vi "File handler.vi"(1 "Path in":path, 2 "Default file name":string, 3 "Read (F) or write (T)?":bool, 4 "Write new File?":bool, 6 "Extension":string="txt", 7 "With dialog?":bool) -> (14 "Path out":path, 15 "Cancelled?":bool, 16 "Data added?":bool)   [LabVIEW 2020]
doc: "This VI handles file name selections with or without a user interface. Files can be read or written. Path in is the path to the file to read or write. Extension is the file extension for the file to write (e.g. txt, jpg). If Read (F) or write (T) is TRUE, Extension must be given and entry must not have a dot. If With dialog? is TRUE, in every case a dialog box will pop up where the file to read or write can be selected. Default file name is used for naming suggestions if a dialog pops up. If Read (F) or write (T)? is TRUE and Write new file? is TRUE, a dialog box will pop up if the selected file name already exists. If Write new file? is FALSE and the selected file name already exists, a dialog box will pop up to ask if data should be added. Data added? indicates if data was added to an existing file. Cancelled? indicates if the user has cancelled the operation. Path out is NotAPath if operation was cancelled or not successful and contains the selected path for the file which was read or written if the operation was successful."
panel:
  # "This vi handles file name selections with or without a user interface.\nFor file writing, \"Extension\" must be given and entry must not have a dot.\nSee manual or VI description for more information."
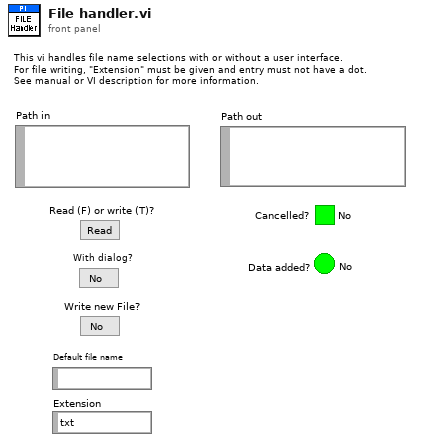
[diagram p1: front panel]
types:
  T1 = enum32{"existing file", "new file", "new or existing file", "existing dir", "new dir", "new or existing dir", "existing file (use LLBs)", "new file (use LLBs)", "new or existing file (use LLBs)", "new or existing file or directory (use LLBs)"}
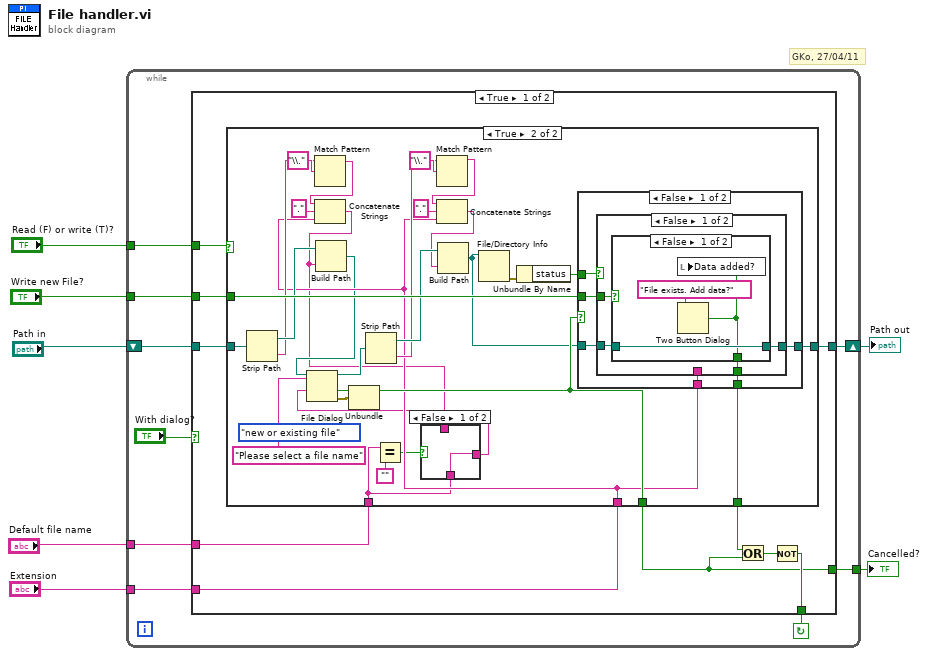
[diagram p0: block diagram]
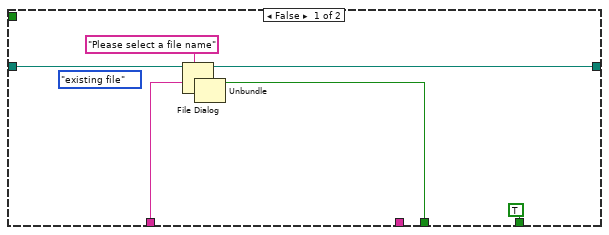
[diagram p2: hidden frame]
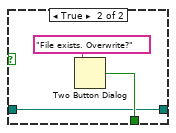
[diagram p4: hidden frame]
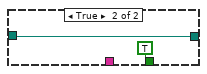
[diagram p5: hidden frame]
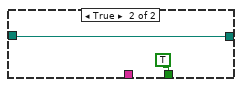
[diagram p6: hidden frame]
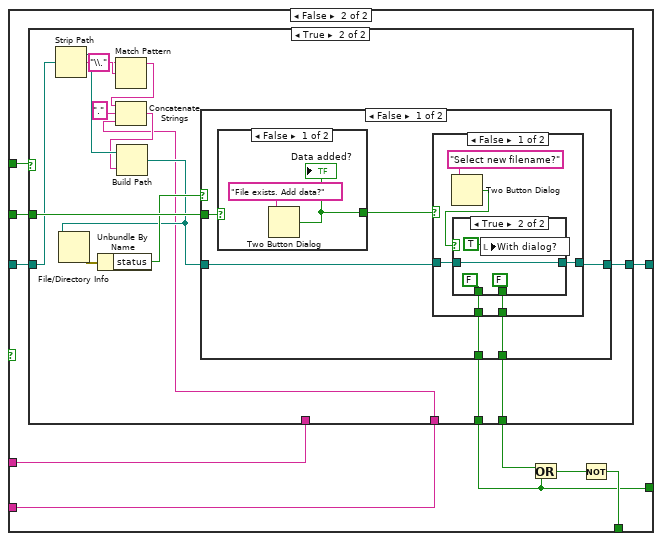
[diagram p7: hidden frame]
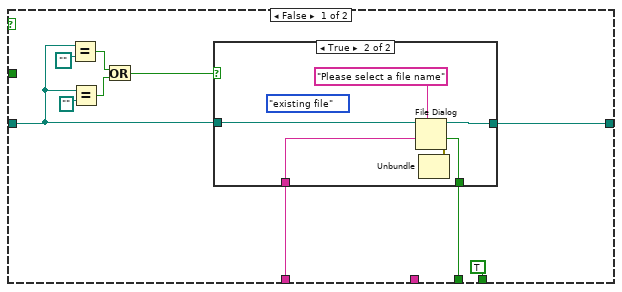
[diagram p8: hidden frame]
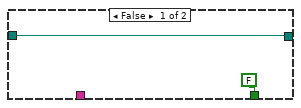
[diagram p9: hidden frame]
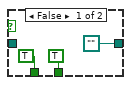
[diagram p10: hidden frame]
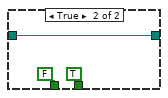
[diagram p11: hidden frame]
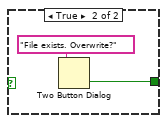
[diagram p12: hidden frame]
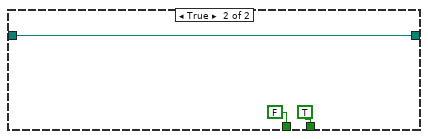
[diagram p13: hidden frame]
diagram:
  # "GKo, 27/04/11"
  n1 = while {
    tunnel: "Extension" -> [w9]
    shift-left: "Path in" -> [w10]
    shift-right: [w11] -> w3
    tunnel: "Default file name" -> [w12]
    tunnel: "Read (F) or write (T)?" -> [w14]
    tunnel: "Write new File?" -> [w15]
    tunnel: [w13] -> w6
    stop <- w16 continue-if-true
    n2 = case shown="True" "With dialog?" {
      tunnel: [w24 w92] -> w16
      tunnel: w15 -> [w23 w91]
      tunnel: w14 -> [w22 w90]
      tunnel: [w18 w86] -> w13
      tunnel: [w21 w89] -> w11
      tunnel: w10 -> [w19 w87]
      tunnel: w12 -> [w20 w88]
      tunnel: w9 -> [w17 w85]
      frame True {
        n3 = case shown="True" w22 {
          tunnel: [TRUE ("T button?") w62] -> w26
          tunnel: w23 -> [_ w61]
          tunnel: [w32 w58] -> w18
          tunnel: [w30 w60] -> w21
          tunnel: w20 -> [w29 w36]
          tunnel: w19 -> [w31 w52]
          tunnel: w17 -> [_ w44]
          frame False {
            (unwired) T1."existing file" ("select mode (2)")
            n4 = File Dialog(7:"Please select a file name" ("prompt"), 9:w29, 11:w31) -> (0:w27:errorcluster, 1:w32:bool, 3:w30:path)  [unwired: 1 in, 4 out]
            n5 = Unbundle(w27) -> ()  [unwired: 3 out]
          }
          frame True {
            (unwired) T1."new or existing file" ("select mode (2)")
            n6 = Strip Path(path=w52) -> (stripped path=w56:path, name=w55:string)
            n7 = Match Pattern(string=w55, regular expression="\\." ("search char (-)")) -> (before substring=w54:string)  [unwired: 4 out]
            n8 = Concatenate Strings(w54, "." ("Substring"), w44) -> (w37:string)
            n9 = Build Path(base path=w56, name or relative path=w37) -> (appended path=w43:path)
            n10 = Equal?(x=w36, y="") -> (x = y?=w38:bool)
            n11 = case shown="False" w38 {
              tunnel: [w63 w64] -> w35
              tunnel: w37 -> [_ w64]
              tunnel: w36 -> [w63 _]
              frame False {
              }
              frame True {
              }
            }
            n12 = File Dialog(7:"Please select a file name" ("prompt"), 9:w35, 11:w43) -> (0:w34:errorcluster, 1:w58:bool, 3:w47:path)  [unwired: 1 in, 4 out]
            n13 = Unbundle(w34) -> ()  [unwired: 3 out]
            n14 = Strip Path(path=w47) -> (stripped path=w50:path, name=w49:string)
            n15 = Match Pattern(string=w49, regular expression="\\." ("search char (-)")) -> (before substring=w46:string)  [unwired: 4 out]
            n16 = Concatenate Strings(w46, "." ("Substring"), w44) -> (w45:string)
            n17 = Build Path(base path=w50, name or relative path=w45) -> (appended path=w42:path)
            n18 = File/Directory Info(path=w42) -> (error out=w41:errorcluster)  [unwired: 1 in, 6 out]
            n19 = Unbundle By Name(w41) -> ("status"=w40:bool)
            n20 = case shown="False" w58 {
              tunnel: [w70 TRUE ("T button?")] -> w62
              tunnel: w61 -> [w69 _]
              tunnel: w40 -> [w68 _]
              tunnel: w42 -> [w67 w83]
              tunnel: [w66 w83] -> w60
              tunnel: w44 -> [w65 _]
              frame False {
                n21 = case shown="False" w68 {
                  tunnel: [w74 TRUE] -> w70
                  tunnel: w69 -> [w73 _]
                  tunnel: w67 -> [w71 w81]
                  tunnel: [w72 w81] -> w66
                  tunnel: w65 -> [_ _]
                  frame False {
                    n22 = case shown="False" w73 {
                      tunnel: [w75 w79] -> w74
                      tunnel: [w76 w78] -> w72
                      tunnel: w71 -> [w76 w78]
                      frame False {
                        n23 = Two Button Dialog(message="File exists. Add data?") -> (T button?=w75:bool)  [unwired: 2 out]
                        n24 = local write "Data added?"(w75) -> ()
                      }
                      frame True {
                        n25 = Two Button Dialog(message="File exists. Overwrite?") -> (T button?=w79:bool)  [unwired: 2 out]
                      }
                    }
                  }
                  frame True {
                  }
                }
              }
              frame True {
              }
            }
          }
        }
        n26 = Or(x=w26, y=w18) -> (x .or. y?=w25:bool)
        n27 = Not(x=w25) -> (.not. x?=w24:bool)
      }
      frame False {
        n28 = case shown="True" w90 {
          tunnel: [TRUE ("T button?") w127] -> w94
          tunnel: w91 -> [_ w126]
          tunnel: [w104 w115] -> w86
          tunnel: [w103 w125] -> w89
          tunnel: w88 -> [w102 _]
          tunnel: w87 -> [w98 w118]
          tunnel: w85 -> [_ w113]
          frame False {
            n29 = Equal?(x=w98, y=path "") -> (x = y?=w96:bool)
            n30 = Equal?(x=w98, y=path "") -> (x = y?=w97:bool)
            n31 = Or(x=w96, y=w97) -> (x .or. y?=w95:bool)
            n32 = case shown="True" w95 {
              tunnel: [FALSE ("cancelled") w111] -> w104
              tunnel: [w106 w110] -> w103
              tunnel: w102 -> [_ w109]
              tunnel: w98 -> [w106 w108]
              frame False {
              }
              frame True {
                (unwired) T1."existing file" ("select mode (2)")
                n33 = File Dialog(7:"Please select a file name" ("prompt"), 9:w109, 11:w108) -> (0:w107:errorcluster, 1:w111:bool, 3:w110:path)  [unwired: 1 in, 4 out]
                n34 = Unbundle(w107) -> ()  [unwired: 3 out]
              }
            }
          }
          frame True {
            n35 = Strip Path(path=w118) -> (stripped path=w123:path, name=w122:string)
            n36 = Match Pattern(string=w122, regular expression="\\." ("search char (-)")) -> (before substring=w121:string)  [unwired: 4 out]
            n37 = Concatenate Strings(w121, "." ("Substring"), w113) -> (w120:string)
            n38 = Build Path(base path=w123, name or relative path=w120) -> (appended path=w114:path)
            n39 = File/Directory Info(path=w114) -> (error out=w117:errorcluster)  [unwired: 1 in, 6 out]
            n40 = Unbundle By Name(w117) -> ("status"=w116:bool)
            n41 = case shown="False" w116 {
              tunnel: [w130 TRUE ("T button?")] -> w127
              tunnel: w126 -> [w133 _]
              tunnel: [w128 w154] -> w125
              tunnel: [w129 FALSE ("T button?")] -> w115
              tunnel: w114 -> [w131 w154]
              frame False {
                n42 = case shown="False" w133 {
                  tunnel: [w150 w152] -> w132
                  frame False {
                    n43 = Two Button Dialog(message="File exists. Add data?") -> (T button?=w150:bool)  [unwired: 2 out]
                    "Data added?" <- w150
                  }
                  frame True {
                    n44 = Two Button Dialog(message="File exists. Overwrite?") -> (T button?=w152:bool)  [unwired: 2 out]
                  }
                }
                n45 = case shown="False" w132 {
                  tunnel: w131 -> [w136 w149]
                  tunnel: [w137 w149] -> w128
                  tunnel: [w135 TRUE] -> w130
                  tunnel: [w134 FALSE] -> w129
                  frame False {
                    n46 = Two Button Dialog(message="Select new filename?") -> (T button?=w138:bool)  [unwired: 2 out]
                    n47 = case shown="True" w138 {
                      tunnel: [path "" ("appended path") w146] -> w137
                      tunnel: w136 -> [_ w146]
                      tunnel: [TRUE FALSE] -> w135
                      tunnel: [TRUE FALSE] -> w134
                      frame False {
                      }
                      frame True {
                        n48 = local write "With dialog?"(TRUE ("With dialog")) -> ()
                      }
                    }
                  }
                  frame True {
                  }
                }
              }
              frame True {
              }
            }
          }
        }
        n49 = Or(x=w94, y=w86) -> (x .or. y?=w93:bool)
        n50 = Not(x=w93) -> (.not. x?=w92:bool)
      }
    }
  }
  "Path out" <- w3
  "Cancelled?" <- w6
